vi "WFGenerate01DC.vi"(7 "Repetitions":T1={"Delay (s)"=0.0, "Interval (s)"=0.0, "Repeat"=1} {"Interval (s)" min=0.0; "Delay (s)" min=0.0}, 8 "error in (no error)":errorcluster, 9 "Waveform Properties":T3={"Fs (Hz)"=20000.0, "Amplitude (V)"=5.0, "Ramp (s)"=0.0, "Duration (s)"=0.1} {"Ramp (s)" min=0.0; "Fs (Hz)" min=0.0}, 10 "Waveform Parameters":T2) -> (0 "error out":errorcluster, 3 "Waveform Out":waveform(dbl)={"t0"=timestamp(0 s since 1904-01-01), "dt"=5e-05, "Y"=array[2000 elements]})   [LabVIEW 2009]
panel:
  out "Waveform Graph":waveform(dbl)(graph)={"t0"=timestamp(0 s since 1904-01-01), "dt"=5e-05, "Y"=array[2000 elements]}
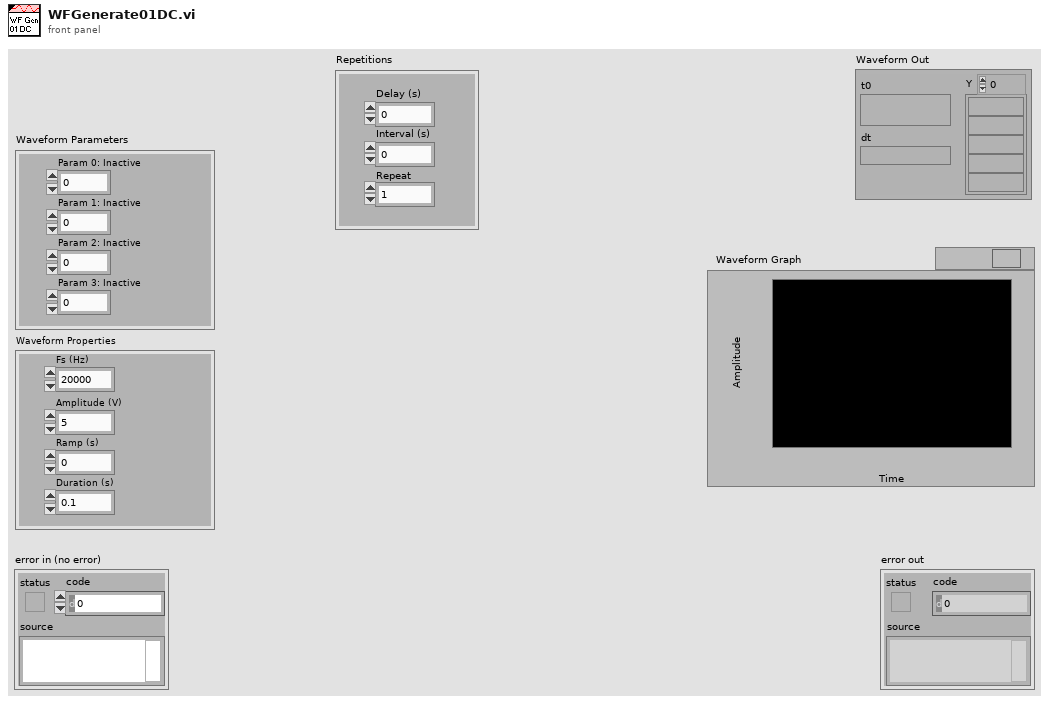
[diagram p1: front panel]
types:
  T1 = cluster{"Delay (s)":dbl, "Interval (s)":dbl, "Repeat":i32}
  T2 = cluster{"Param 0: Inactive":dbl, "Param 1: Inactive":dbl, "Param 2: Inactive":dbl, "Param 3: Inactive":dbl}
  T3 = cluster{"Fs (Hz)":dbl, "Amplitude (V)":dbl, "Ramp (s)":dbl, "Duration (s)":dbl}
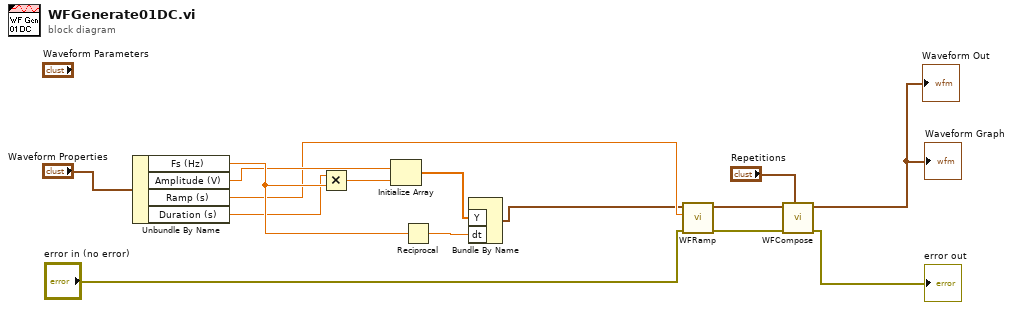
[diagram p0: block diagram]
diagram:
  n1 = Unbundle By Name("Waveform Properties") -> ("Fs (Hz)"=w13:dbl, "Amplitude (V)"=w12:dbl, "Ramp (s)"=w3:dbl, "Duration (s)"=w9:dbl)
  n2 = Multiply(x=w9, y=w13) -> (x*y=w11:dbl)
  n3 = Initialize Array(w12, w11) -> (w10:dbl[])
  n4 = Reciprocal(x=w13) -> (1/x=w15:dbl)
  n5 = Bundle By Name("Y"=w10, "dt"=w15) -> (w1:waveform(dbl))  [unwired: 1 in]
  n6 = call "WFRamp.vi"("error in (no error)"="error in (no error)", "Ramp Length (s)"=w3, "Waveform In"=w1) -> ("error out"=w5:errorcluster, "Waveform Out"=w2:waveform(dbl))  [unwired: 7 in]
  n7 = call "WFCompose.vi"("Repetitions"="Repetitions", "error in (no error)"=w5, "Waveform In"=w2) -> ("error out"=→"error out":errorcluster, "Analog Waveform Out"=→"Waveform Out" →"Waveform Graph":waveform(dbl))  [unwired: 7 in]
